vi "Configure Socket Protocol Mode.vi"(8 "error in (no error)":errorcluster, 9 "Protocol Mode (Raw)":i32(ring) items=["Raw", "Agilent", "IEEE1147"], 10 "Channel (1)":i32=1, 11 "VISA resource name":refnum<visa-resource-name>) -> (0 "error out":errorcluster, 3 "VISA resource name out":refnum<visa-resource-name>)   [LabVIEW 2020, in "Rohde&Schwarz CMXP Base.lvlib"]
doc: "Sets the protocol operation mode for direct socket communication.\n\nAttribute:\nRSCMXPBASE_ATTR_SOCKET_PROTOCOL_MODE\n\nRemote-control command:\nSYSTem:COMMunicate:SOCKet<i>:MODE"
uses:
  <instrlib>/Rohde&Schwarz CMXP Base/Rohde&Schwarz CMXP Base.lvlib
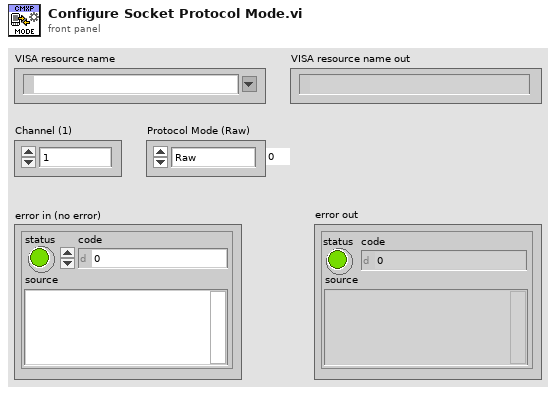
[diagram p1: front panel]
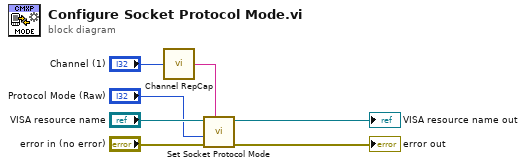
[diagram p0: block diagram]
diagram:
  n1 = call <instrlib>:"Channel RepCap.vi"("Channel In"="Channel (1)") -> ("Channel Out"=w2:string)  [unwired: 1 out]
  n2 = call "Set Socket Protocol Mode"("Repeated Capabilities"=w2, "error in (no error)"="error in (no error)", "Socket Protocol Mode (0 - Raw)"="Protocol Mode (Raw)", "instrument handle"="VISA resource name") -> ("error out"=→"error out":errorcluster, "instrument handle out"=→"VISA resource name out":refnum<visa-resource-name>)  [unwired: 6 in]
